vi "Assign Correction Table To RX.vi"(8 "error in (no error)":errorcluster, 9 "Correction Tables (\"Table1\")":string[](array[string]), 10 "Signal Path (\"RF1.1\")":string="RF1.1", 11 "VISA resource name":refnum<visa-resource-name>) -> (0 "error out":errorcluster, 3 "VISA resource name out":refnum<visa-resource-name>)   [LabVIEW 2015, in "Rohde&Schwarz CMXP Base.lvlib"]
doc: "Assigns one or more correction tables to the RX direction of a signal path. If there is an existing assignment, it is overwritten.\n\nThe directions refer to the test instrument (RX of the instrument).\n\nAttribute:\n-\n\nRemote-control command:\n[CONFigure:]TENVironment:SPATh:CTABle:RX"
uses:
  <instrlib>/Rohde&Schwarz CMXP Base/Rohde&Schwarz CMXP Base.lvlib
  <instrlib>/Rohde&Schwarz CMXP Base/Private/rsidr_core.llb/rsidr_core.lvlib
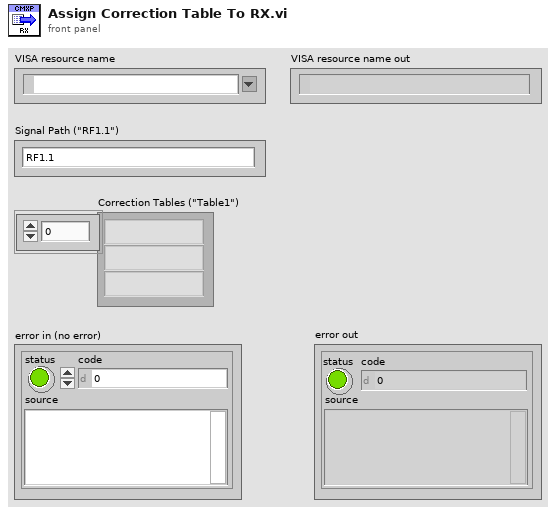
[diagram p1: front panel]
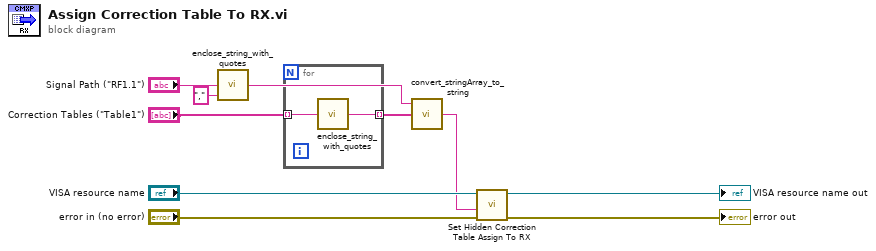
[diagram p0: block diagram]
diagram:
  n1 = call <instrlib>:"enclose_string_with_quotes.vi"("String after"=",", "String to enclose"="Signal Path (\"RF1.1\")") -> ("String out"=w6:string)  [unwired: 3 in]
  n2 = for {
    tunnel: "Correction Tables (\"Table1\")" -> [w12] mode=indexing
    tunnel: [w11] -> w5 mode=indexing
    n3 = call <instrlib>:"enclose_string_with_quotes.vi"("String to enclose"=w12) -> ("String out"=w11:string)  [unwired: 4 in]
  }
  n4 = call <instrlib>:"convert_stringArray_to_string.vi"("string array in"=w5, "String to add before (\"\")"=w6) -> ("string out"=w2:string)  [unwired: 3 in]
  n5 = call "Set Hidden Correction Table Assign To RX"("error in (no error)"="error in (no error)", "Hidden Correction Table Assign To RX ()"=w2, "instrument handle"="VISA resource name") -> ("error out"=→"error out":errorcluster, "instrument handle out"=→"VISA resource name out":refnum<visa-resource-name>)  [unwired: 7 in]
